vi "CIEncoder.vi"(8 "error in (no error)":errorcluster, 11 "reference":refnum<k24>) -> (0 "error out":errorcluster, 1 "PulsesPerRevolution":i32, 2 "Units":i32(ring) items=["Degrees", "Radians", "Ticks"], 3 "reference out":refnum<k24>, 4 "InitialAngle":dbl, 5 "ZIndexMode":i32(ring) items=["Disabled"=0, "LatchCounter"=8, "ResetCounter"=32], 6 "DecodingType":i32(ring) items=["X1", "X2", "X4"])   [LabVIEW 2009]
uses:
  C:/Program Files/National Instruments/LabVIEW 2009/vi.lib/ULx/ULx_LV.dll
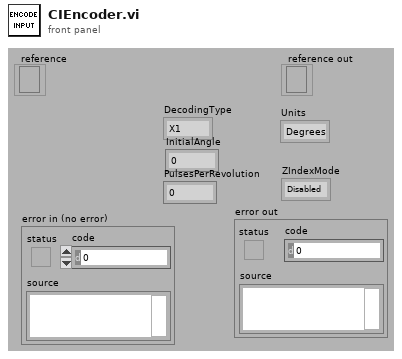
[diagram p1: front panel]
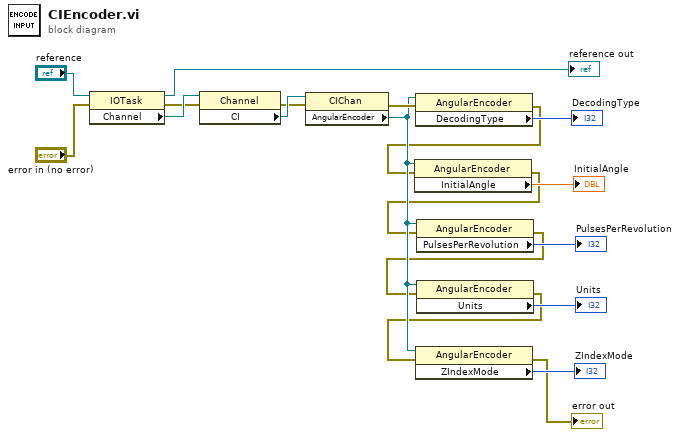
[diagram p0: block diagram]
diagram:
  n1 = property class="IOTask"(reference="reference", error in="error in (no error)") -> (reference out=→"reference out":refnum<k24>, error out=w17:errorcluster, "Channel"=w19:refnum<k24>)
  n2 = property class="Channel"(reference=w19, error in=w17) -> (error out=w15:errorcluster, "CI"=w16:refnum<k24>)  [unwired: 1 out]
  n3 = property class="CIChan"(reference=w16, error in=w15) -> (error out=w14:errorcluster, "AngularEncoder"=w10:refnum<k24>)  [unwired: 1 out]
  n4 = property class="AngularEncoder"(reference=w10, error in=w14) -> (error out=w5:errorcluster, "DecodingType"=→"DecodingType":i32)  [unwired: 1 out]
  n5 = property class="AngularEncoder"(reference=w10, error in=w5) -> (error out=w4:errorcluster, "InitialAngle"=→"InitialAngle":dbl)  [unwired: 1 out]
  n6 = property class="AngularEncoder"(reference=w10, error in=w4) -> (error out=w3:errorcluster, "PulsesPerRevolution"=→"PulsesPerRevolution":i32)  [unwired: 1 out]
  n7 = property class="AngularEncoder"(reference=w10, error in=w3) -> (error out=w2:errorcluster, "Units"=→"Units":i32)  [unwired: 1 out]
  n8 = property class="AngularEncoder"(reference=w10, error in=w2) -> (error out=→"error out":errorcluster, "ZIndexMode"=→"ZIndexMode":i32)  [unwired: 1 out]
